vi "Obtain Gate Reference.vi"(0 "name (unnamed)":string, 2 "create if not found? (T)":bool=TRUE, 3 "error in (no error)":errorcluster) -> (7 "gate":T1, 9 "created new?":bool, 10 "error out":errorcluster)   [LabVIEW 2015, in "Gates.lvlib"]
doc: "Obtains a reference to an existing gate or creates a new gate and returns a reference to that gate."
uses:
  Gates.lvlib
  Gate.ctl
  Gate Pass.ctl
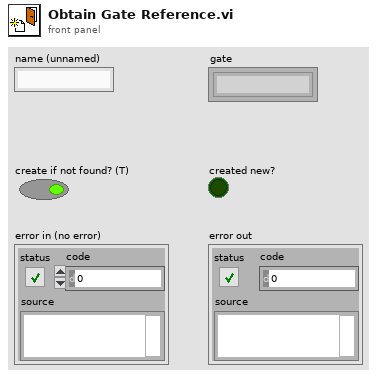
[diagram p1: front panel]
types:
  T1 = typedef "Gates.lvlib/Gate.ctl" = refnum<k1>
  T2 = typedef "Gates.lvlib/Gate Pass.ctl" = refnum<k1>
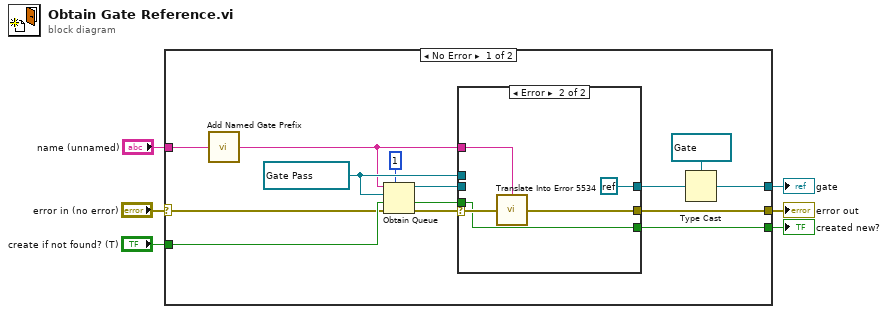
[diagram p0: block diagram]
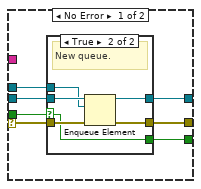
[diagram p2: hidden frame]
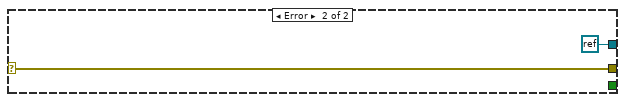
[diagram p4: hidden frame]
diagram:
  n1 = case shown="No Error" "error in (no error)" {
    selector: "error in (no error)" -> [w11 w43]
    tunnel: "name (unnamed)" -> [w20 _]
    tunnel: "create if not found? (T)" -> [w19 _]
    tunnel: [w14 _] -> w4
    tunnel: [w10 w43] -> w2
    tunnel: [w9 refnum<k0> refnum] -> w1
    frame No Error {
      w13 = T1 refnum items=["Gate"] ("Data Log File Refnum")
      w15 = T2 refnum items=["Gate Pass"] ("Data Log File Refnum")
      n2 = call "Add Named Gate Prefix.vi"("name in"=w20) -> ("name out"=w7:string)
      n3 = Obtain Queue(max queue size (-1, unlimited)=1, name (unnamed)=w7, element data type=w15, create if not found? (T)=w19, error in (no error)=w11) -> (queue out=w16:refnum<queue>, created new?=w17:bool, error out=w18:errorcluster)
      n4 = case shown="Error" w18 {
        selector: w18 -> [w26 w41]
        tunnel: w17 -> [w27 w38]
        tunnel: w16 -> [w25 _]
        tunnel: [w24 w40] -> w10
        tunnel: w15 -> [w23 _]
        tunnel: [w22 w38] -> w14
        tunnel: [w21 refnum<k0> refnum] -> w12
        tunnel: w7 -> [_ w37]
        frame No Error {
          n5 = case shown="True" w27 {
            selector: w27 -> [w28 w31]
            tunnel: w26 -> [w29 w35]
            tunnel: w25 -> [w30 w36]
            tunnel: [w29 w34] -> w24
            tunnel: [w30 w32] -> w21
            tunnel: w23 -> [_ w33]
            tunnel: [w28 w31] -> w22
            frame False {
              # "Obtained existing queue."
            }
            frame True {
              # "New queue."
              n6 = Enqueue Element(queue=w36, element=w33, error in (no error)=w35) -> (queue out=w32:refnum<queue>, error out=w34:errorcluster)  [unwired: 1 in, 1 out]
            }
          }
        }
        frame Error {
          n7 = call "Translate Into Error 5534.vi"("error in (no error)"=w41, "name"=w37) -> ("error out"=w40:errorcluster)
        }
      }
      n8 = Type Cast(type=w13, x=w12) -> (*(type *) &x=w9:T1)
    }
    frame Error {
    }
  }
  "error out" <- w2
  "created new?" <- w4
  "gate" <- w1
